vi "Get Status.vi"(8 "error in (no error)":errorcluster, 11 "State in":refnum<class "State.lvclass">) -> (0 "error out":errorcluster, 2 "Status":string, 3 "State out":refnum<class "State.lvclass">)   [LabVIEW 2013, in "State.lvclass"]
uses:
  State.lvclass
  State.lvclass/State.ctl
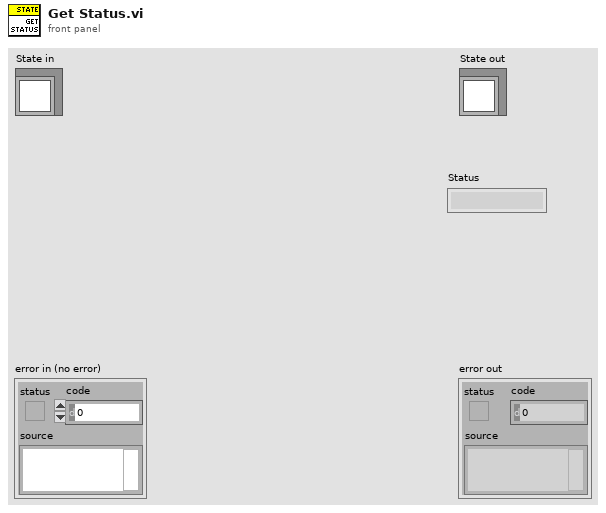
[diagram p1: front panel]
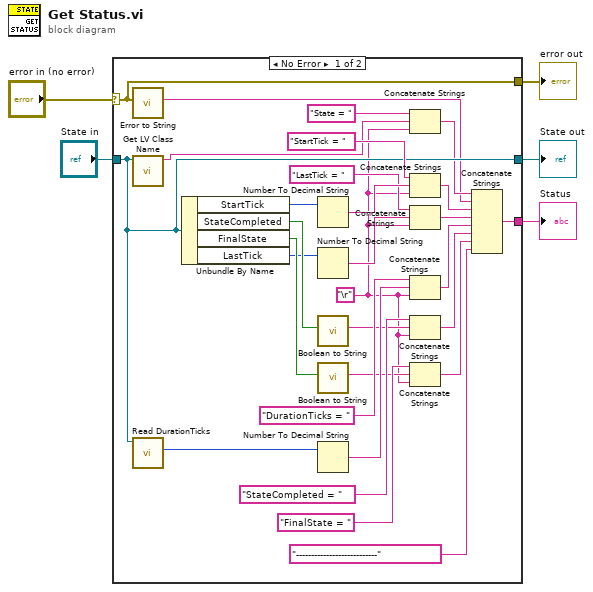
[diagram p0: block diagram]
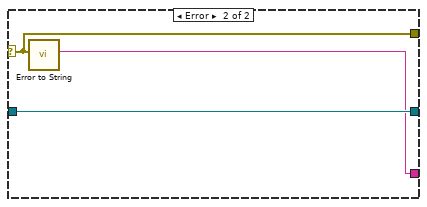
[diagram p2: hidden frame]
diagram:
  n1 = case shown="No Error" "error in (no error)" {
    selector: "error in (no error)" -> [w23 w36]
    tunnel: [w23 w36] -> w4
    tunnel: [w28 w37] -> w2
    tunnel: "State in" -> [w28 w37]
    tunnel: [w7 w35] -> w1
    frame No Error {
      w15 = "\r"
      n2 = call "Error to String.vi"("error in (no error)"=w23) -> ("String out"=w13:string)  [unwired: 10 in]
      n3 = call <vilib>:"Get LV Class Name.vi"("object"=w28) -> ("class name"=w26:string)  [unwired: 9 in, 1 out]
      n4 = call "Read DurationTicks.vi"("State in"=w28) -> ("DurationTicks"=w31:u32)  [unwired: 8 in, 2 out]
      n5 = Unbundle By Name(w28) -> ("StartTick"=w34:u32, "StateCompleted"=w22:bool, "FinalState"=w20:bool, "LastTick"=w18:u32)
      n6 = Number To Decimal String(number=w34) -> (decimal integer string=w32:string)  [unwired: 1 in]
      n7 = Number To Decimal String(number=w18) -> (decimal integer string=w16:string)  [unwired: 1 in]
      n8 = call "Boolean to String.vi"("Boolean"=w22) -> ("String"=w21:string)  [unwired: 10 in]
      n9 = call "Boolean to String.vi"("Boolean"=w20) -> ("String"=w19:string)  [unwired: 10 in]
      n10 = Number To Decimal String(number=w31) -> (decimal integer string=w29:string)  [unwired: 1 in]
      n11 = Concatenate Strings("State = ", w26, w15) -> (w14:string)
      n12 = Concatenate Strings("StartTick = ", w32, w15) -> (w12:string)
      n13 = Concatenate Strings("LastTick = ", w16, w15) -> (w11:string)
      n14 = Concatenate Strings("DurationTicks = ", w29, w15) -> (w10:string)
      n15 = Concatenate Strings("StateCompleted = ", w21, w15) -> (w9:string)
      n16 = Concatenate Strings("FinalState = ", w19, w15) -> (w8:string)
      n17 = Concatenate Strings(w14, w13, w12, w11, w10, w9, w8, "---------------------------") -> (w7:string)
    }
    frame Error {
      n18 = call "Error to String.vi"("error in (no error)"=w36) -> ("String out"=w35:string)  [unwired: 10 in]
    }
  }
  "error out" <- w4
  "State out" <- w2
  "Status" <- w1
